vi "Initialize.vi"(8 "error in (no error)":errorcluster, 11 "ASIA Pump C Settings in":T1 {"channel" min=-1 max=1 step=1; "ASIA Pump #" min=0 step=1}) -> (0 "error out":errorcluster, 1 "Initialized":bool, 2 "No Pump Connected":bool=TRUE, 3 "ASIA Pump C Settings out":T1)   [LabVIEW 2018, in "ASIA Pump.lvlib"]
uses:
  ASIA Pump.lvlib
  Pump Settings.ctl
  Program Files (x86)/Pfizer/FAST/data/AsiaPumpInterface.dll
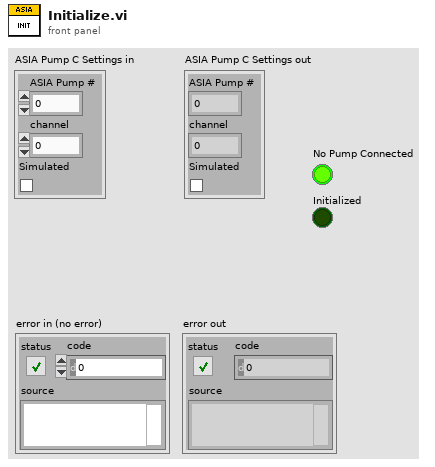
[diagram p1: front panel]
types:
  T1 = typedef "ASIA Pump.lvlib/Pump Settings.ctl" = cluster{"ASIA Pump #":i32, "channel":i32, "Simulated":bool}
  T2 = cluster{"Busy":bool, "PumpCnt":dbl, "RemoteEntered":bool, "OverpressureSet":bool}[]
  T3 = cluster{"Busy":bool, "PumpCnt":dbl, "RemoteEntered":bool, "OverpressureSet":bool}
  T4 = enum16{"Error", "Uninitialised", "Initialising", "Idle", "Filling", "Full", "Emptying", "Empty", "Pumping", "Default"}
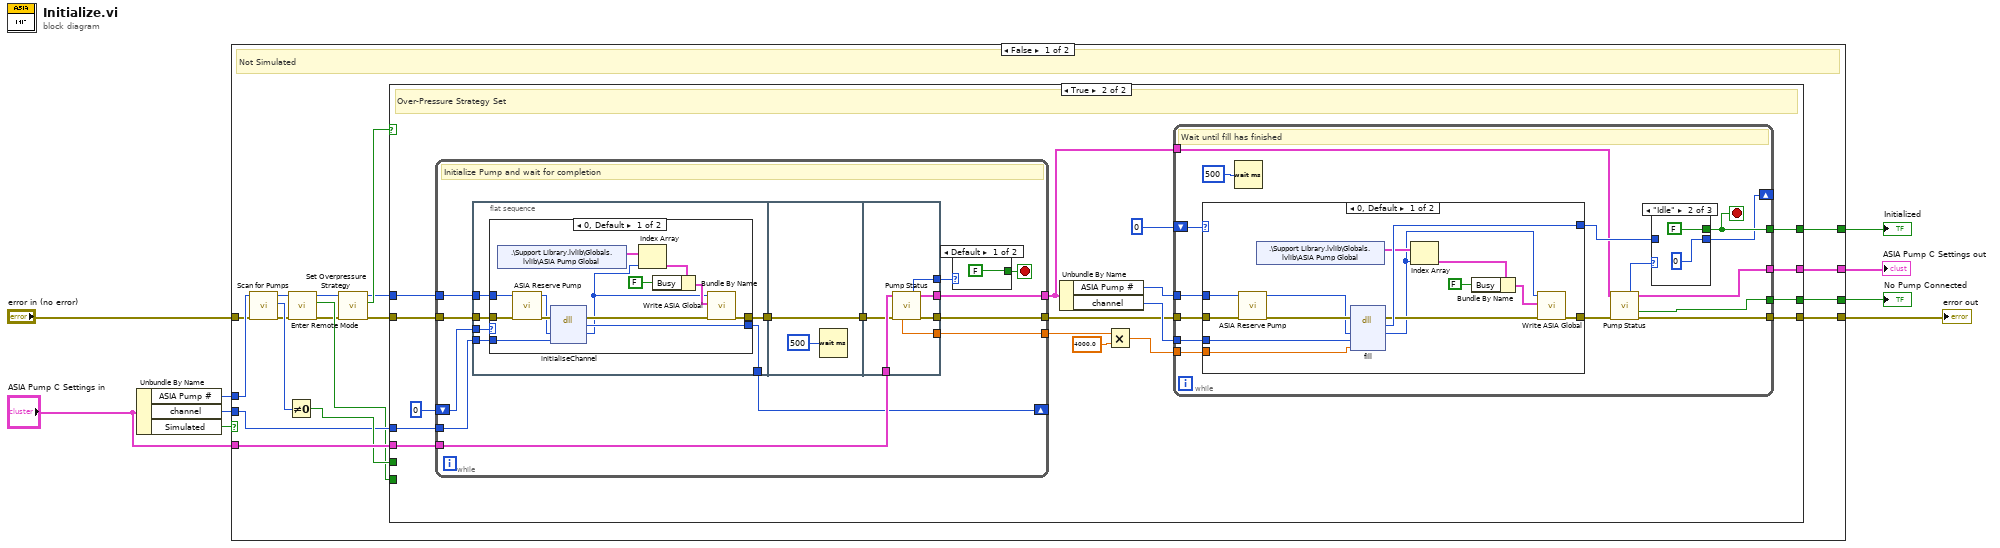
[diagram p0: block diagram]
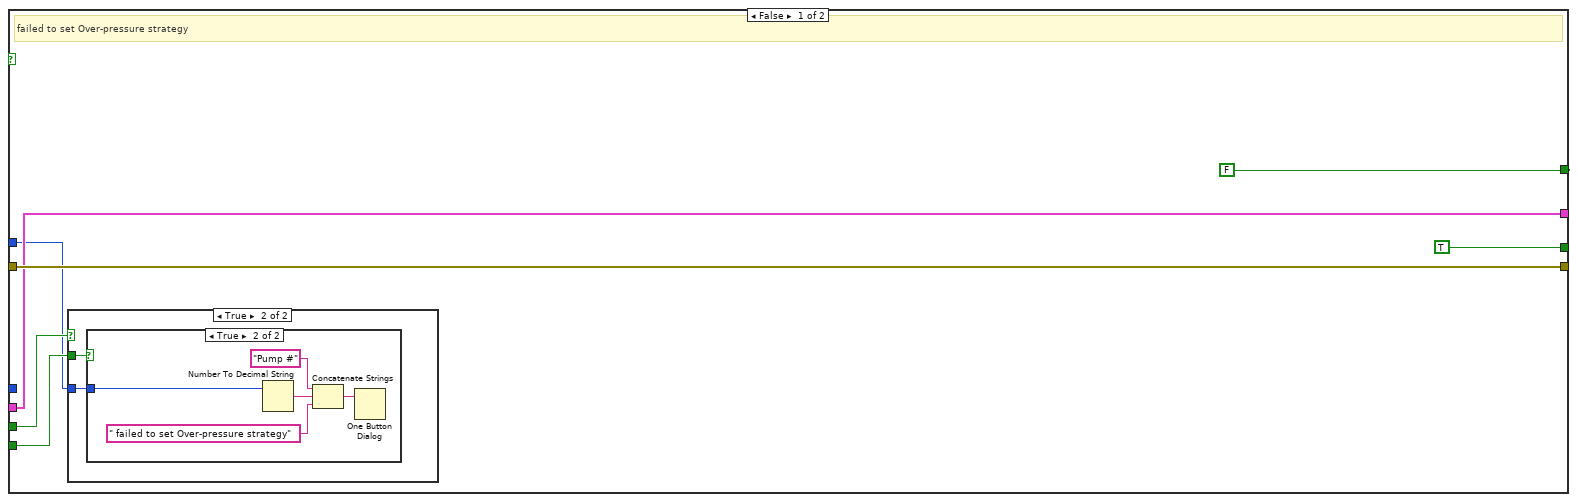
[diagram p2: hidden frame]
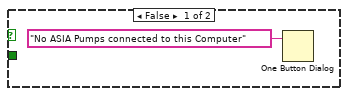
[diagram p3: hidden frame]
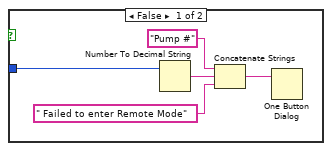
[diagram p4: hidden frame]
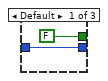
[diagram p6: hidden frame]
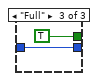
[diagram p7: hidden frame]
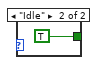
[diagram p9: hidden frame]
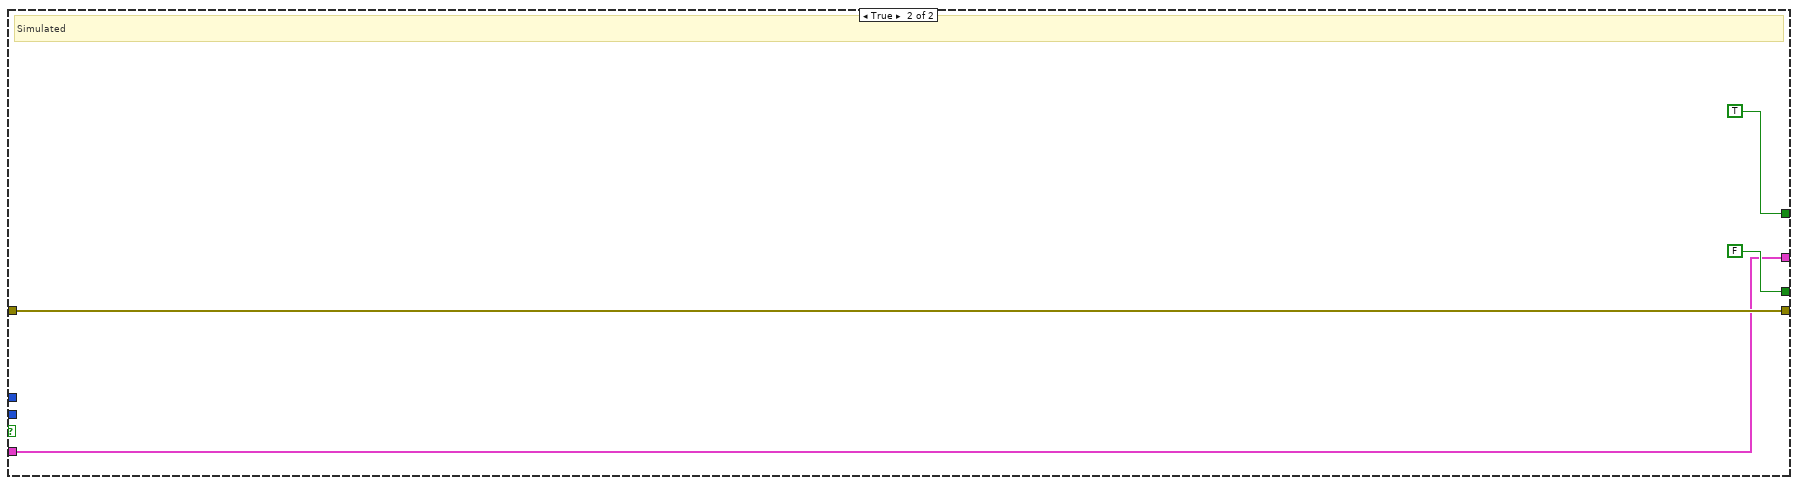
[diagram p10: hidden frame]
diagram:
  n1 = Unbundle By Name("ASIA Pump C Settings in") -> ("ASIA Pump #"=w1:i32, "channel"=w3:i32, "Simulated"=w2:bool)
  n2 = case shown="False" w2 {
    tunnel: "error in (no error)" -> [w19 w149]
    tunnel: [w27 w149] -> w9
    tunnel: w3 -> [w21 _]
    tunnel: [w26 FALSE] -> w8
    tunnel: "ASIA Pump C Settings in" -> [w25 w146]
    tunnel: [w24 TRUE] -> w7
    tunnel: [w22 w146] -> w6
    tunnel: w1 -> [w20 _]
    frame False {
      # "Not Simulated"
      n3 = call "Scan for Pumps.vi"("error in (no error)"=w19, "ASIA Pump #"=w20) -> ("error out"=w15:errorcluster, "pumpCnt"=w18:u32, "ASIA Pump #"=w16:i32)  [unwired: 7 in]
      n4 = Not Equal To 0?(x=w18) -> (x != 0?=w23:bool)
      n5 = call "Enter Remote Mode.vi"("error in (no error)"=w15, "ASIA Pump #"=w16) -> ("error out"=w13:errorcluster, "Completed"=w17:bool, "ASIA Pump #"=w14:i32)  [unwired: 7 in]
      n6 = call "Set Overpressure Strategy.vi"("error in (no error)"=w13, "ASIA Pump #"=w14) -> ("error out"=w11:errorcluster, "strategySet"=w12:bool, "ASIA Pump #"=w10:i32)  [unwired: 7 in]
      n7 = case shown="True" w12 {
        tunnel: w11 -> [w33 w63]
        tunnel: [TRUE w51] -> w26
        tunnel: [w33 w52] -> w27
        tunnel: w10 -> [w28 w60]
        tunnel: w25 -> [w29 w61]
        tunnel: [FALSE w50] -> w24
        tunnel: w23 -> [w31 _]
        tunnel: w17 -> [w30 _]
        tunnel: w21 -> [_ w59]
        tunnel: [w29 w48] -> w22
        frame False {
          # "failed to set Over-pressure strategy"
          n8 = case shown="True" w31 {
            tunnel: w30 -> [_ w37]
            tunnel: w28 -> [_ w36]
            frame False {
              n9 = One Button Dialog(message="No ASIA Pumps connected to this Computer") -> ()  [unwired: 1 in, 1 out]
            }
            frame True {
              n10 = case shown="True" w37 {
                tunnel: w36 -> [w38 w43]
                frame False {
                  n11 = Number To Decimal String(number=w38) -> (decimal integer string=w41:string)  [unwired: 1 in]
                  n12 = Concatenate Strings("Pump #" ("string"), w41, " Failed to enter Remote Mode" ("message")) -> (w42:string)
                  n13 = One Button Dialog(message=w42) -> ()  [unwired: 1 in, 1 out]
                }
                frame True {
                  n14 = Number To Decimal String(number=w43) -> (decimal integer string=w46:string)  [unwired: 1 in]
                  n15 = Concatenate Strings("Pump #" ("string"), w46, " failed to set Over-pressure strategy" ("message")) -> (w47:string)
                  n16 = One Button Dialog(message=w47) -> ()  [unwired: 1 in, 1 out]
                }
              }
            }
          }
        }
        frame True {
          # "Over-Pressure Strategy Set"
          n17 = while {
            tunnel: [w107] -> w54
            tunnel: w63 -> [w113]
            tunnel: [w106] -> w53
            tunnel: w60 -> [w112]
            tunnel: w59 -> [w111]
            tunnel: w61 -> [w108]
            tunnel: [w104] -> w58
            shift-right: [w103] -> _
            shift-left: u8 0 ("Bool") -> [w102]
            stop <- w114 stop-if-true
            # "Initialize Pump and wait for completion"
            n18 = flat-sequence {
              tunnel: w113 -> [w120]
              tunnel: w112 -> [w118]
              tunnel: w111 -> [w117]
              tunnel: [w119] -> w110
              tunnel: [w116] -> w103
              tunnel: w102 -> [w115]
              tunnel: w110 -> [w137]
              tunnel: [w137] -> w109
              tunnel: w109 -> [w142]
              tunnel: w108 -> [w143]
              tunnel: [w141] -> w107
              tunnel: [w140] -> w106
              tunnel: [w139] -> w105
              tunnel: [w138] -> w104
              frame #0 {
                n19 = case shown="0, Default" w115 {
                  selector: w115 -> [_ w134]
                  tunnel: w120 -> [w131 w135]
                  tunnel: [w126 w135] -> w119
                  tunnel: w118 -> [w129 _]
                  tunnel: w117 -> [w133 _]
                  tunnel: [w132 w134] -> w116
                  frame 0, Default {
                    n20 = shared-variable ".\\Support Library.lvlib\\Globals.lvlib\\ASIA Pump Global"() -> (w123:T2)  [unwired: 1 in, 1 out]
                    n21 = call "ASIA Reserve Pump.vi"("error in (no error)"=w131, "ASIA Pump #"=w129) -> ("error out"=w130:errorcluster, "ASIA Pump #"=w128:i32)  [unwired: 8 in]
                    n22 = dll-call lib="C:/Program Files (x86)/Pfizer/FAST/data/AsiaPumpInterface.dll" fn="initialiseChannel"(error in=w130, "pumpNum"=w128, "channel"=w133) -> (error out=w127:errorcluster, "Bool"=w132:u8, "pumpNum"=w121:u32)  [unwired: 3 in, 1 out]
                    n23 = Index Array(array=w123, index=w121) -> (element=w122:T3)
                    n24 = Bundle By Name(cluster=w122, "Busy"=FALSE) -> (w124:T3)
                    n25 = call "Write ASIA Global.vi"("error in (no error)"=w127, "ASIA Global"=w124, "Pump Number"=w121) -> ("error out"=w126:errorcluster)  [unwired: 7 in, 1 out]
                  }
                  frame 1 {
                  }
                }
              }
              frame #1 {
                n26 = Wait (ms)(milliseconds to wait=u32 500) -> ()  [unwired: 1 out]
              }
              frame #2 {
                n27 = call "Pump Status.vi"("ASIA Pump C Settings in"=w143, "error in (no error)"=w142) -> ("PumpStatusCode"=w139:T4, "ASIA Pump C Settings out"=w140:T1, "syringeSize (ml)"=w138:sgl, "error out"=w141:errorcluster)  [unwired: 5 in, 5 out]
              }
            }
            n28 = case shown="Default" w105 {
              tunnel: [FALSE TRUE] -> w114
              frame Default {
              }
              frame "Idle" {
              }
            }
          }
          n29 = Unbundle By Name(w53) -> ("ASIA Pump #"=w56:i32, "channel"=w55:i32)
          n30 = Multiply(x=w58, y=4000.0) -> (x*y=w57:dbl)
          n31 = while {
            tunnel: [w69] -> w52
            tunnel: w53 -> [w68]
            tunnel: w54 -> [w78]
            tunnel: w56 -> [w77]
            tunnel: w55 -> [w76]
            tunnel: w57 -> [w75]
            tunnel: [w74] -> w50
            tunnel: [w65] -> w51
            shift-right: [w71] -> _
            shift-left: u8 0 ("Bool") -> [w73]
            tunnel: [w66] -> w48
            stop <- w74 stop-if-true
            # "Wait until fill has finished"
            n32 = case shown="0, Default" w73 {
              selector: w73 -> [_ w94]
              tunnel: w78 -> [w89 w95]
              tunnel: w77 -> [w90 _]
              tunnel: w76 -> [w93 _]
              tunnel: w75 -> [w92 _]
              tunnel: [w86 w95] -> w70
              tunnel: [w91 w94] -> w72
              frame 0, Default {
                n33 = call "ASIA Reserve Pump.vi"("error in (no error)"=w89, "ASIA Pump #"=w90) -> ("error out"=w88:errorcluster, "ASIA Pump #"=w80:i32)  [unwired: 8 in]
                n34 = shared-variable ".\\Support Library.lvlib\\Globals.lvlib\\ASIA Pump Global"() -> (w83:T2)  [unwired: 1 in, 1 out]
                n35 = dll-call lib="C:/Program Files (x86)/Pfizer/FAST/data/AsiaPumpInterface.dll" fn="fill"(error in=w88, "pumpNum"=w80, "channel"=w93, "rate"=w92) -> (error out=w87:errorcluster, "Bool"=w91:u8, "pumpNum"=w81:u32)  [unwired: 4 in, 1 out]
                n36 = Index Array(array=w83, index=w81) -> (element=w82:T3)
                n37 = Bundle By Name(cluster=w82, "Busy"=FALSE) -> (w84:T3)
                n38 = call "Write ASIA Global.vi"("error in (no error)"=w87, "ASIA Global"=w84, "Pump Number"=w81) -> ("error out"=w86:errorcluster)  [unwired: 7 in, 1 out]
              }
              frame 1 {
              }
            }
            n39 = Wait (ms)(milliseconds to wait=u32 500) -> ()  [unwired: 1 out]
            n40 = call "Pump Status.vi"("ASIA Pump C Settings in"=w68, "error in (no error)"=w70) -> ("PumpStatusCode"=w67:T4, "ASIA Pump C Settings out"=w66:T1, "Connection Error"=w65:bool, "error out"=w69:errorcluster)  [unwired: 5 in, 5 out]
            n41 = case shown="\"Idle\"" w67 {
              tunnel: [FALSE FALSE TRUE] -> w74
              tunnel: w72 -> [w96 _ w100]
              tunnel: [w96 0 w100] -> w71
              frame Default {
              }
              frame "Idle" {
              }
              frame "Full" {
              }
            }
          }
        }
      }
    }
    frame True {
      # "Simulated"
    }
  }
  "error out" <- w9
  "ASIA Pump C Settings out" <- w6
  "No Pump Connected" <- w8
  "Initialized" <- w7
